vi "Read Sample From Container.vi"(6 "Queue timeout in ms (-1)":i32=-1, 8 "error in (no error)":errorcluster, 9 "Read from SHV (F)":bool, 11 "Container":T1) -> (0 "error out":errorcluster, 1 "Queue timed out?":bool, 2 "Sample out":refnum<class "Sample.lvclass">, 3 "Container":T1, 4 "Overflow Sample":refnum<class "Sample.lvclass">)   [LabVIEW 2015, in "Sample.lvclass"]
uses:
  Sample.lvclass
  Controls/Sample Container.ctl
  Sample.lvclass/Sample.ctl
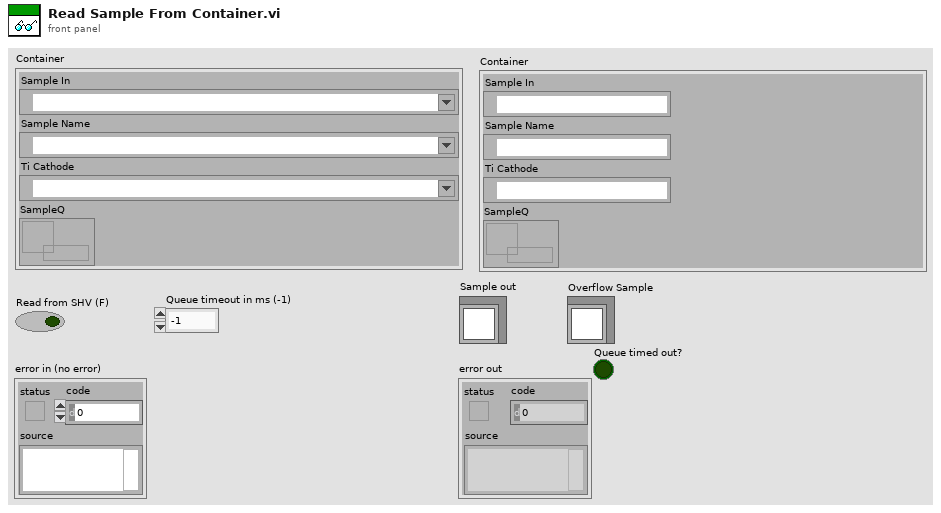
[diagram p1: front panel]
types:
  T1 = typedef "Sample Container.ctl" = cluster{"Sample In":refnum<k21>, "Sample Name":refnum<k21>, "Ti Cathode":refnum<k21>, "SampleQ":refnum<queue>}
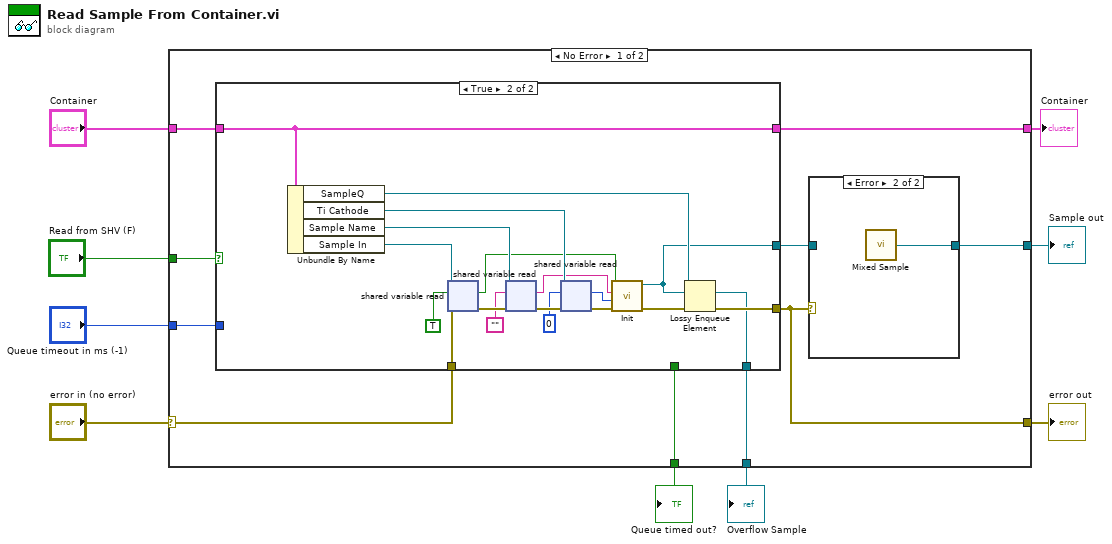
[diagram p0: block diagram]
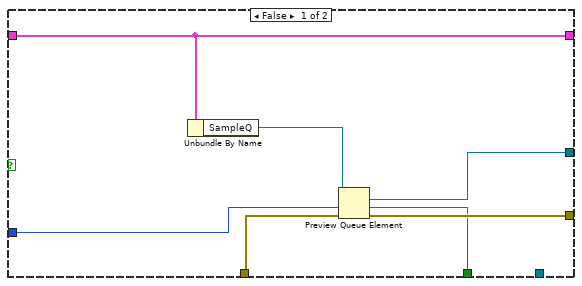
[diagram p2: hidden frame]
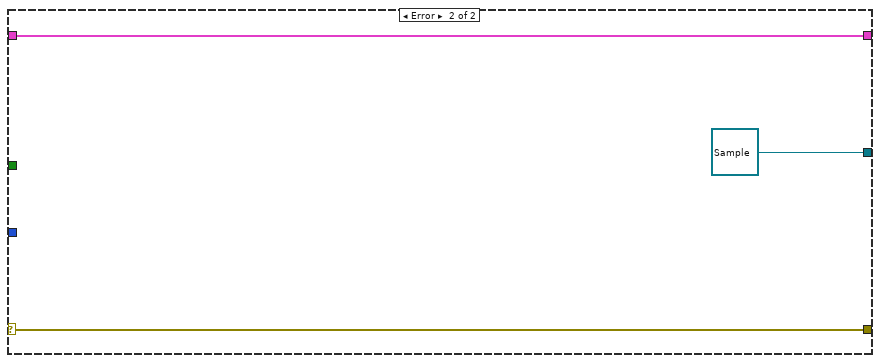
[diagram p4: hidden frame]
diagram:
  n1 = case shown="No Error" "error in (no error)" {
    selector: "error in (no error)" -> [w12 w50]
    tunnel: [w15 w50] -> w8
    tunnel: [w19 refnum<class "Sample.lvclass"> refnum ("Sample in")] -> w6
    tunnel: "Container" -> [w18 w48]
    tunnel: [w14 w48] -> w5
    tunnel: "Read from SHV (F)" -> [w16 _]
    tunnel: [w13 _] -> w3
    tunnel: "Queue timeout in ms (-1)" -> [w11 _]
    tunnel: [w10 _] -> w1
    frame No Error {
      n2 = case shown="True" w16 {
        tunnel: w18 -> [w23 w33]
        tunnel: [w25 w29] -> w17
        tunnel: [w24 w31] -> w15
        tunnel: w12 -> [w22 w43]
        tunnel: [w23 w33] -> w14
        tunnel: [_ w28] -> w13
        tunnel: w11 -> [w21 _]
        tunnel: [w20 _] -> w10
        frame False {
          n3 = Unbundle By Name(w23) -> ("SampleQ"=w26:refnum<queue>)
          n4 = Preview Queue Element(queue=w26, timeout in ms (-1)=w21, error in (no error)=w22) -> (element=w25:refnum<class "Sample.lvclass">, timed out?=w20:bool, error out=w24:errorcluster)  [unwired: 1 out]
        }
        frame True {
          n5 = Unbundle By Name(w33) -> ("SampleQ"=w30:refnum<queue>, "Ti Cathode"=w39:refnum<k21>, "Sample Name"=w41:refnum<k21>, "Sample In"=w27:refnum<k21>)
          n6 = shared-variable-read(w27, w43, TRUE) -> (w45:errorcluster, w35:bool)  [unwired: 2 out]
          n7 = shared-variable-read(w41, w45, "") -> (w44:errorcluster, w34:string)  [unwired: 2 out]
          n8 = shared-variable-read(w39, w44, i8 0 ("Ti Cathode")) -> (w37:errorcluster, w36:i8)  [unwired: 2 out]
          n9 = call "Init.vi"("error in (no error)"=w37, "Ti Cathode"=w36, "Name"=w34, "Sample in"=w35) -> ("error out"=w32:errorcluster, "Sample out"=w29:refnum<class "Sample.lvclass">)  [unwired: 6 in]
          n10 = Lossy Enqueue Element(queue=w30, element=w29, error in (no error)=w32) -> (overflow element=w28:refnum<class "Sample.lvclass">, error out=w31:errorcluster)  [unwired: 2 out]
        }
      }
      n11 = case shown="Error" w15 {
        tunnel: [w46 w47] -> w19
        tunnel: w17 -> [w46 _]
        frame No Error {
        }
        frame Error {
          n12 = call "Mixed Sample.vi"() -> ("Mixed Sample (Sample In: true)"=w47:refnum<class "Sample.lvclass">)
        }
      }
    }
    frame Error {
    }
  }
  "error out" <- w8
  "Sample out" <- w6
  "Container" <- w5
  "Overflow Sample" <- w3
  "Queue timed out?" <- w1
